vi "Asynchronous Call and Collect.vi"() -> ()   [LabVIEW 2023]
doc: "This VI demonstrates an asynchronous call and collecting the outputs later.\n\nWhen this VI is run, it asynchronously calls a target VI and will wait for the results in a different location. \n\nThis example uses the Start Asynchronous Call method and the Open VI Reference option 0x100."
panel:
  out "Elapsed Time (s)":dbl format="%.1g"
  out "X + Y":dbl
  in  "Y":dbl=2.0
  in  "X":dbl=1.0
  # "Overview: Demonstrates the use of the call and collect option (0x100) with Asynchronous VI Calls.\nInstructions:\nRun the VI. Observe the behavior of the VI being called asynchronously. See the block diagram for more information."
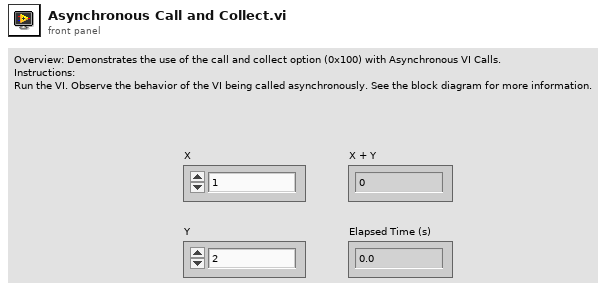
[diagram p1: front panel]
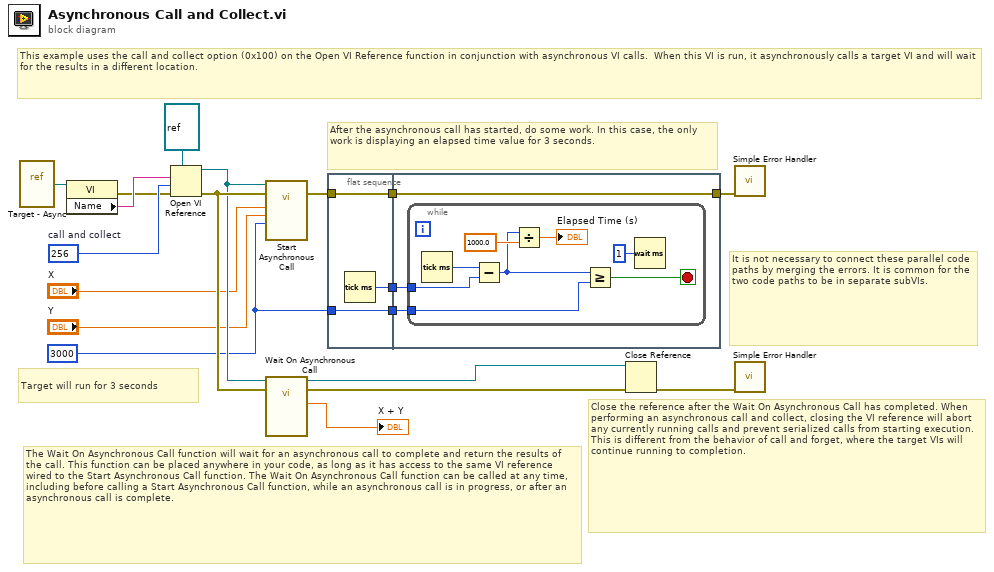
[diagram p0: block diagram]
diagram:
  w1 = u32 3000 ("Wait (Milliseconds)")
  w19 = 256  # call and collect
  # "This example uses the call and collect option (0x100) on the Open VI Reference function in conjunction with asynchronous VI calls.  When this VI is run, it asynchronously calls a target VI and will wait for the results in a different location."
  # "It is not necessary to connect these parallel code paths by merging the errors. It is common for the two code paths to be in separate subVIs."
  # "Close the reference after the Wait On Asynchronous Call has completed. When performing an asynchronous call and collect, closing the VI reference will abort any currently running calls and prevent serialized calls from starting execution. This is different from the behavior of call and forget, where the target VIs will continue running to completion."
  # "After the asynchronous call has started, do some work. In this case, the only work is displaying an elapsed time value for 3 seconds."
  # "The Wait On Asynchronous Call function will wait for an asynchronous call to complete and return the results of the call. This function can be placed anywhere in your code, as long as it has access to the same VI reference wired to the Start Asynchronous Call function. The Wait On Asynchronous Call function can be called at any time, including before calling a Start Asynchronous Call function, while an asynchronous call is in progress, or after an asynchronous call is complete."
  # "Target will run for 3 seconds"
  n1 = vi-ref "Target - Async.vi"() -> (w14:refnum<vi>)
  n2 = property class="VI"(reference=w14) -> (error out=w5:errorcluster, "Name"=w13:string)  [unwired: 1 in, 1 out]
  n3 = Open VI Reference(type specifier VI Refnum (for type only)=refnum<vi> refnum, vi path=w13, options=w19, error in (no error)=w5) -> (vi reference=w11:refnum<vi>, error out=w12:errorcluster)  [unwired: 2 in]
  n4 = call-by-ref "Start Asynchronous Call"(reference=w11, error in=w12, "Wait (ms)"=w1, "Y"="Y", "X"="X") -> (error out=w10:errorcluster)  [unwired: 8 in, 2 out]
  n5 = call-by-ref "Wait On Asynchronous Call"(reference=w11, error in=w12) -> (reference out=w16:refnum<vi>, error out=w15:errorcluster, "X + Y"=→"X + Y":dbl)  [unwired: 11 in]
  n6 = flat-sequence {
    tunnel: w10 -> [w22]
    tunnel: [w22] -> w4
    tunnel: [w21] -> w3
    tunnel: [w20] -> w2
    tunnel: w1 -> [w20]
    tunnel: [w23] -> w9
    tunnel: w4 -> [w23]
    tunnel: w3 -> [w25]
    tunnel: w2 -> [w24]
    frame #0 {
      n7 = Tick Count (ms)() -> (millisecond timer value=w21:u32)
    }
    frame #1 {
      n8 = while {
        tunnel: w25 -> [w30]
        tunnel: w24 -> [w28]
        stop <- w29 stop-if-true
        n9 = Tick Count (ms)() -> (millisecond timer value=w27:u32)
        n10 = Subtract(x=w27, y=w30) -> (x-y=w26:u32)
        n11 = Divide(x=w26, y=1000.0) -> (x/y=→"Elapsed Time (s)":dbl)
        n12 = Greater Or Equal?(x=w26, y=w28) -> (x >= y?=w29:bool)
        n13 = Wait (ms)(milliseconds to wait=u32 1) -> ()  [unwired: 1 out]
      }
    }
  }
  n14 = Close Reference(reference=w16, error in (no error)=w15) -> (error out=w17:errorcluster)
  n15 = call <vilib>:"Simple Error Handler.vi"("error in (no error)"=w9) -> ()  [unwired: 4 in, 5 out]
  n16 = call <vilib>:"Simple Error Handler.vi"("error in (no error)"=w17) -> ()  [unwired: 4 in, 5 out]
